vi "RT Stop ALL Task.vi"(8 "error in":errorcluster, 11 "Task out":T1={"DI task out"="", "DO task out"="", "TC task out"="", "AI task out"="", "AO task out"="", "AI"=TRUE, "AO"=TRUE, "DI"=TRUE, "DO"=TRUE, "TC"=TRUE}) -> (0 "error out":errorcluster)   [LabVIEW 2022 SP3]
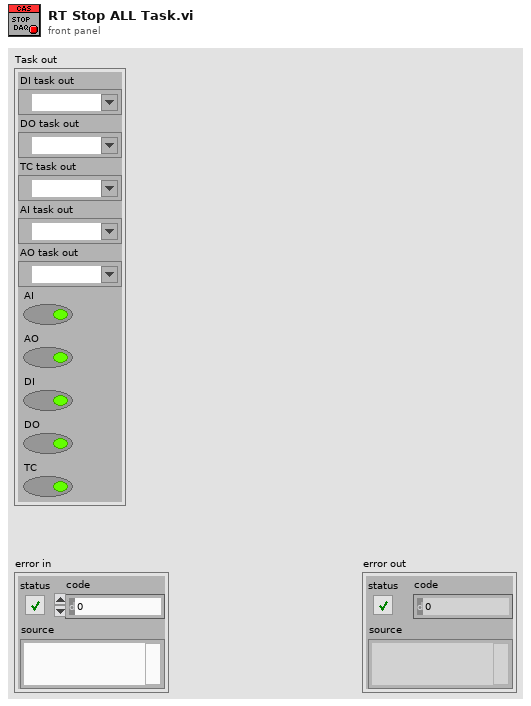
[diagram p1: front panel]
types:
  T1 = cluster{"DI task out":refnum<k21>, "DO task out":refnum<k21>, "TC task out":refnum<k21>, "AI task out":refnum<k21>, "AO task out":refnum<k21>, "AI":bool, "AO":bool, "DI":bool, "DO":bool, "TC":bool}
  T2 = enum16{"AI", "AO", "DI", "DO", "TC", "Strain", "ACC"}[]
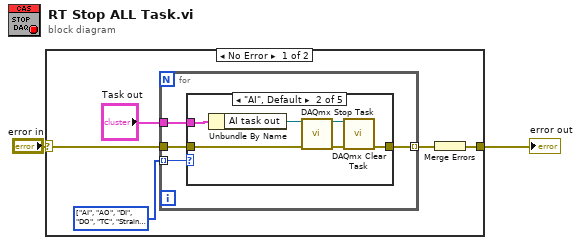
[diagram p0: block diagram]
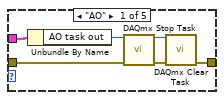
[diagram p2: hidden frame]
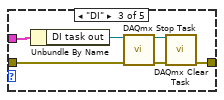
[diagram p3: hidden frame]
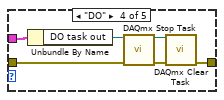
[diagram p4: hidden frame]
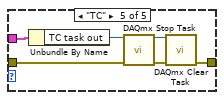
[diagram p5: hidden frame]
diagram:
  n1 = case shown="No Error" "error in" {
    selector: "error in" -> [w7 w42]
    tunnel: [w5 w42] -> w1
    frame No Error {
      w3 = T2 [enum."AI", enum."AO", enum."DI", enum."DO", enum."TC", enum."Strain", enum."ACC"] items=["AI", "AO", "DI", "DO", "TC", "Strain", "ACC"] ("Task List")
      n2 = for {
        tunnel: w7 -> [w11]
        tunnel: [w9] -> w6 mode=indexing
        tunnel: w3 -> [w10] mode=indexing
        tunnel: "Task out" -> [w8]
        n3 = case shown="\"AI\", Default" w10 {
          tunnel: w11 -> [w15 w21 w27 w33 w39]
          tunnel: [w14 w20 w26 w32 w38] -> w9
          tunnel: w8 -> [w13 w19 w25 w31 w37]
          frame "AO" {
            n4 = Unbundle By Name(w13) -> ("AO task out"=w12:refnum<k21>)
            n5 = call <vilib>:"DAQmx Stop Task.vi"("task/channels in"=w12, "error in"=w15) -> ("task out"=w17:refnum<k21>, "error out"=w16:errorcluster)  [unwired: 12 in]
            n6 = call <vilib>:"DAQmx Clear Task.vi"("task in"=w17, "error in"=w16) -> ("error out"=w14:errorcluster)  [unwired: 13 in]
          }
          frame "AI", Default {
            n7 = Unbundle By Name(w19) -> ("AI task out"=w18:refnum<k21>)
            n8 = call <vilib>:"DAQmx Stop Task.vi"("task/channels in"=w18, "error in"=w21) -> ("task out"=w23:refnum<k21>, "error out"=w22:errorcluster)  [unwired: 12 in]
            n9 = call <vilib>:"DAQmx Clear Task.vi"("task in"=w23, "error in"=w22) -> ("error out"=w20:errorcluster)  [unwired: 13 in]
          }
          frame "DI" {
            n10 = Unbundle By Name(w25) -> ("DI task out"=w24:refnum<k21>)
            n11 = call <vilib>:"DAQmx Stop Task.vi"("task/channels in"=w24, "error in"=w27) -> ("task out"=w29:refnum<k21>, "error out"=w28:errorcluster)  [unwired: 12 in]
            n12 = call <vilib>:"DAQmx Clear Task.vi"("task in"=w29, "error in"=w28) -> ("error out"=w26:errorcluster)  [unwired: 13 in]
          }
          frame "DO" {
            n13 = Unbundle By Name(w31) -> ("DO task out"=w30:refnum<k21>)
            n14 = call <vilib>:"DAQmx Stop Task.vi"("task/channels in"=w30, "error in"=w33) -> ("task out"=w35:refnum<k21>, "error out"=w34:errorcluster)  [unwired: 12 in]
            n15 = call <vilib>:"DAQmx Clear Task.vi"("task in"=w35, "error in"=w34) -> ("error out"=w32:errorcluster)  [unwired: 13 in]
          }
          frame "TC" {
            n16 = Unbundle By Name(w37) -> ("TC task out"=w36:refnum<k21>)
            n17 = call <vilib>:"DAQmx Stop Task.vi"("task/channels in"=w36, "error in"=w39) -> ("task out"=w41:refnum<k21>, "error out"=w40:errorcluster)  [unwired: 12 in]
            n18 = call <vilib>:"DAQmx Clear Task.vi"("task in"=w41, "error in"=w40) -> ("error out"=w38:errorcluster)  [unwired: 13 in]
          }
        }
      }
      n19 = Merge Errors(w6) -> (w5:errorcluster)
    }
    frame Error {
    }
  }
  "error out" <- w1
